vi "Shutdown.vi"(8 "error in (no error)":errorcluster, 11 "DemoLasers in":refnum<class "DemoLasers.lvclass">) -> (0 "error out":errorcluster, 3 "DemoLasers out":refnum<class "DemoLasers.lvclass">)   [LabVIEW 2020, in "DemoLasers.lvlib" / "DemoLasers.lvclass"]
uses:
  DemoLasers.lvclass
  Hardware Abstraction Layer/Component/Laser/Laser/Laser.lvclass
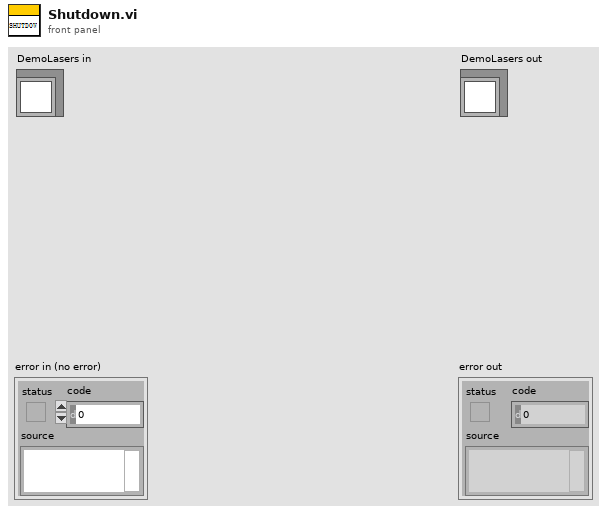
[diagram p1: front panel]
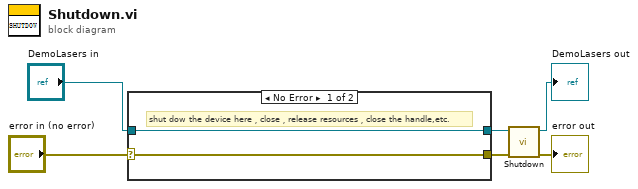
[diagram p0: block diagram]
diagram:
  n1 = case shown="No Error" "error in (no error)" {
    selector: "error in (no error)" -> [w7 w10]
    tunnel: [w7 w10] -> w2
    tunnel: [w8 w9] -> w1
    tunnel: "DemoLasers in" -> [w8 w9]
    frame No Error {
      # "shut dow the device here，close，release resources，close the handle,etc."
    }
    frame Error {
    }
  }
  n2 = call-parent "Shutdown.vi"("error in (no error)"=w2, "GRMActor in"=w1) -> ("error out"=→"error out":errorcluster, "GRMActor out"=→"DemoLasers out":refnum<class "DemoLasers.lvclass">)  [unwired: 8 in]
